vi "System Exec SSID.vi"() -> ()   [LabVIEW 2016]
panel:
  out "after substring":string
  out "match substring":string
  out "standard output":string
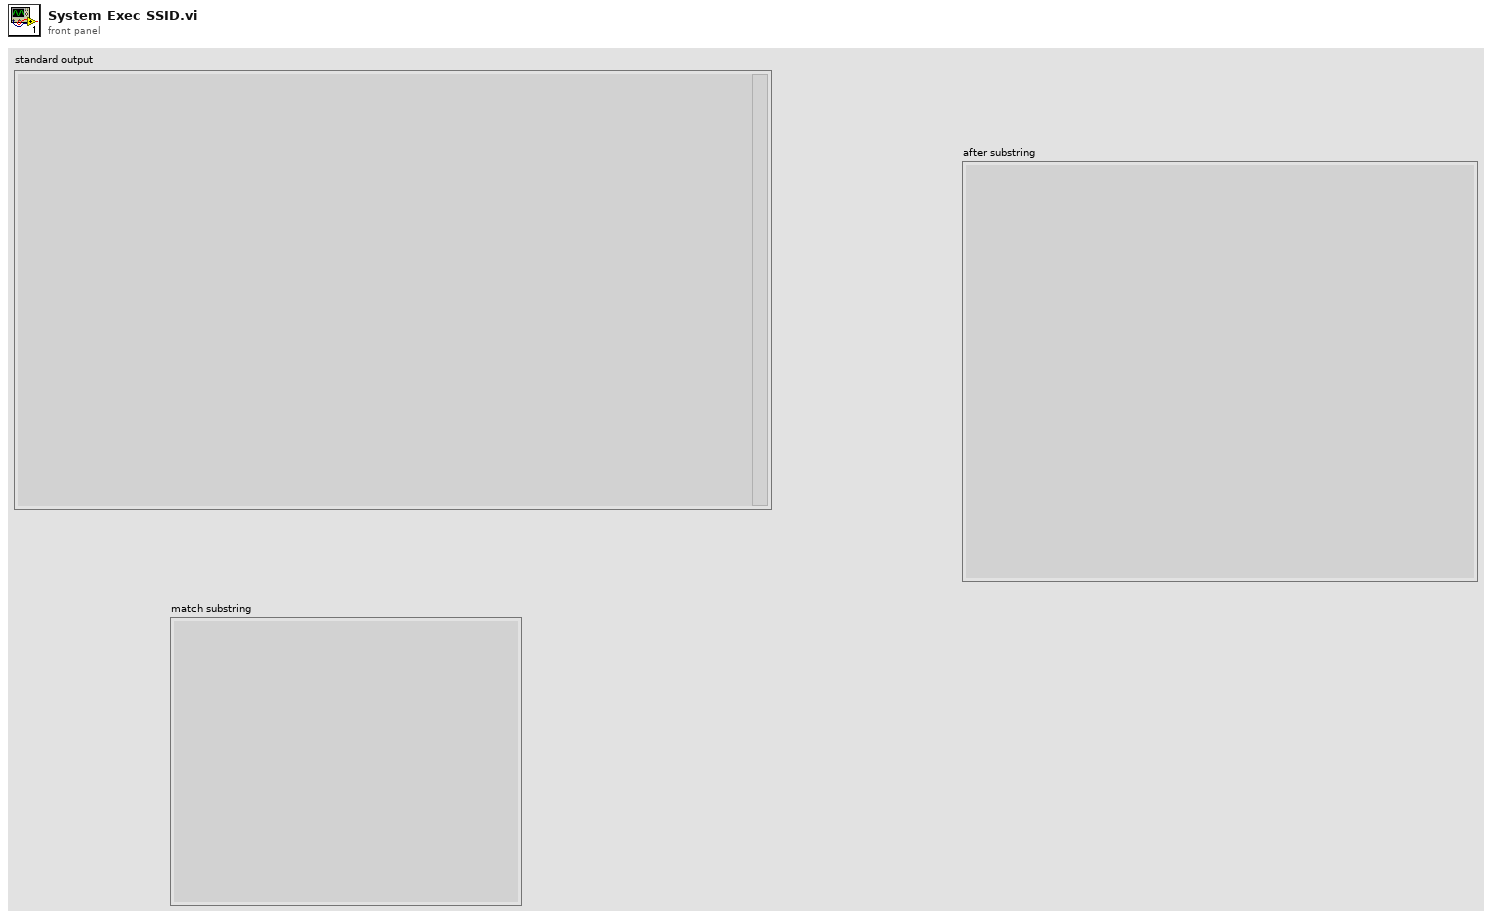
[diagram p1: front panel]
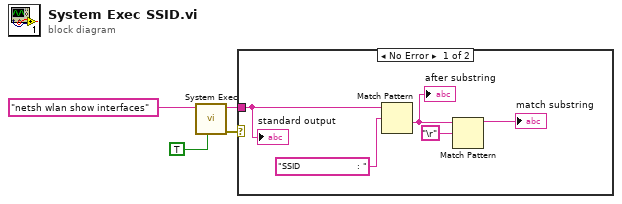
[diagram p0: block diagram]
diagram:
  n1 = call <vilib>:"System Exec.vi"("run minimized? (F)"=TRUE, "command line"="netsh wlan show interfaces") -> ("error out"=w1:errorcluster, "standard output"=w2:string)  [unwired: 6 in, 2 out]
  n2 = case shown="No Error" w1 {
    tunnel: w2 -> [w9 _]
    frame No Error {
      n3 = Match Pattern(string=w9, regular expression="SSID                   : ") -> (after substring=w7:string)  [unwired: 1 in, 3 out]
      "after substring" <- w7
      n4 = Match Pattern(string=w7, regular expression="\r") -> (before substring=→"match substring":string)  [unwired: 1 in, 3 out]
      "standard output" <- w9
    }
    frame Error {
    }
  }
